vi "Read Channel Array.vi"(8 "error in":errorcluster, 10 "channels":refnum<class "Channel.lvclass">[](array[class]), 11 "counter driven output mode in":refnum<class "Counter Driven Output Mode.lvclass">) -> (0 "error out":errorcluster, 2 "channel settings":T1[](array[typedef]), 3 "counter driven output mode out":refnum<class "Counter Driven Output Mode.lvclass">)   [LabVIEW 2017, in "Scan Engine Scripting.lvlib" / "Counter Driven Output Mode.lvclass"]
doc: "Returns the array of channel settings from the channels."
uses:
  Counter Driven Output Mode.lvclass
  Channel Classes/Channel/Channel.lvclass
  Controls/counter driven output channel settings.ctl
  Channel Classes/Counter Driven Output Channel/Counter Driven State.ctl
  Channel Classes/Counter Driven Output Channel/Counter Driven Output Channel.lvclass
  Scan Engine Scripting.lvlib
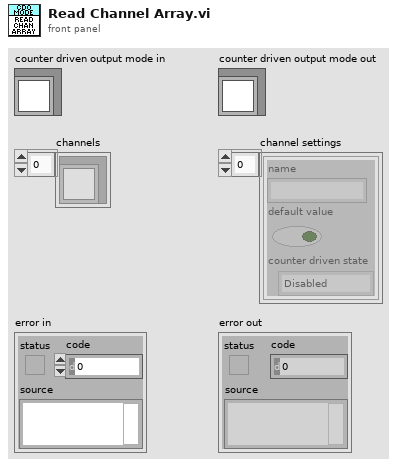
[diagram p1: front panel]
types:
  T1 = typedef "Scan Engine Scripting.lvlib/counter driven output channel settings.ctl" = cluster{"name":string, "default value":bool, "counter driven state":T2}
  T2 = typedef "Scan Engine Scripting.lvlib/Counter Driven Output Channel.lvclass/Counter Driven State.ctl" = enum16{"Disabled", "Enabled"}
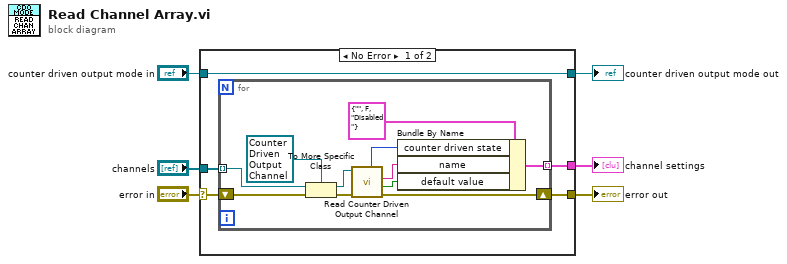
[diagram p0: block diagram]
diagram:
  n1 = case shown="No Error" "error in" {
    selector: "error in" -> [w9 w24]
    tunnel: [w8 w24] -> w5
    tunnel: [w11 w23] -> w3
    tunnel: "counter driven output mode in" -> [w11 w23]
    tunnel: "channels" -> [w10 _]
    tunnel: [w7 _] -> w1
    frame No Error {
      n2 = for {
        tunnel: w10 -> [w15] mode=indexing
        tunnel: [w18] -> w7 mode=indexing
        shift-right: [w22] -> w8
        shift-left: w9 -> [w16]
        n3 = To More Specific Class(target class=refnum<class "Counter Driven Output Channel.lvclass"> refnum ("Scan Engine Scripting.lvlib:Counter Driven Output Channel.lvclass"), reference=w15, error in=w16) -> (specific class reference=w13:refnum<class "Counter Driven Output Channel.lvclass">, error out=w12:errorcluster)
        n4 = call "Read Counter Driven Output Channel.vi"("error in"=w12, "counter driven output channel in"=w13) -> ("error out"=w22:errorcluster, "default value"=w19:bool, "name"=w20:string, "counter driven state"=w17:T2)  [unwired: 4 in, 2 out]
        n5 = Bundle By Name(cluster=T1 {"name"="", "default value"=FALSE, "counter driven state"=enum."Disabled"} ("channel settings"), "counter driven state"=w17, "name"=w20, "default value"=w19) -> (w18:T1)
      }
    }
    frame Error {
    }
  }
  "error out" <- w5
  "counter driven output mode out" <- w3
  "channel settings" <- w1
